vi "test Basic Future Resolution - Error.vi"(8 "error in (no error)":errorcluster, 11 "TestCase in":refnum<class "Futures Tests.lvclass">) -> (0 "error out":errorcluster, 3 "TestCase out":refnum<class "Futures Tests.lvclass">)   [LabVIEW 2017, in "Futures Tests.lvclass"]
uses:
  Futures Tests.lvclass
  <vilib>/Utility/error.llb/Error Cluster From Error Code.vi
  <vilib>/ErrorRing/Error Ring.xnode
  <vilib>/addons/_JKI Toolkits/VI Tester/TestCase.llb/TestCase.lvclass
  Futures/Futures.lvlib
  Futures/Future/Future.lvclass
  Futures/Promise/Promise.lvclass
  C:/Program Files (x86)/National Instruments/LabVIEW 2017/vi.lib/addons/_JKI Toolkits/VI Tester/TestCase.llb/TestCase.lvclass
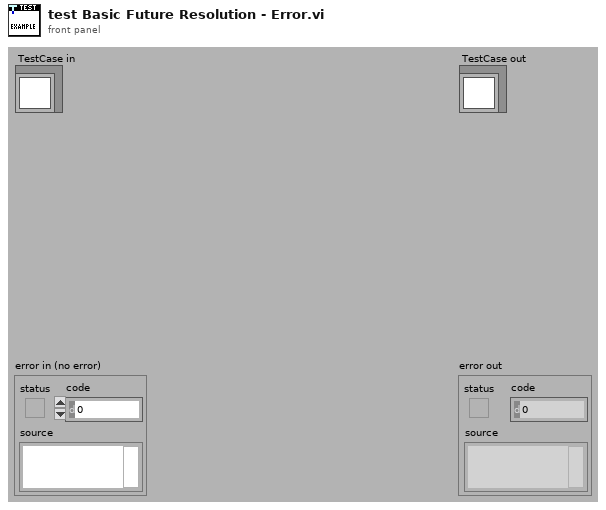
[diagram p1: front panel]
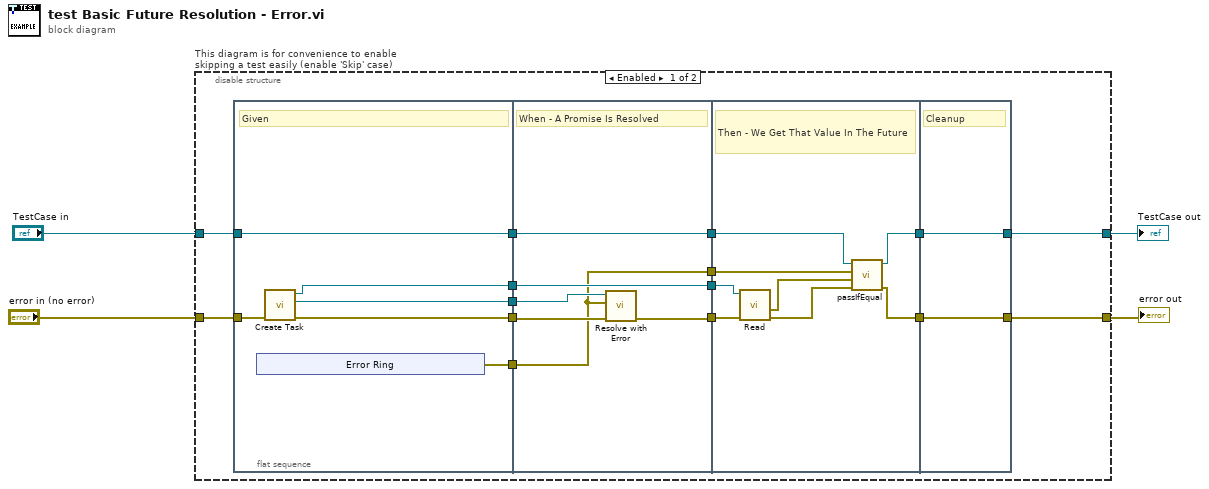
[diagram p0: block diagram]
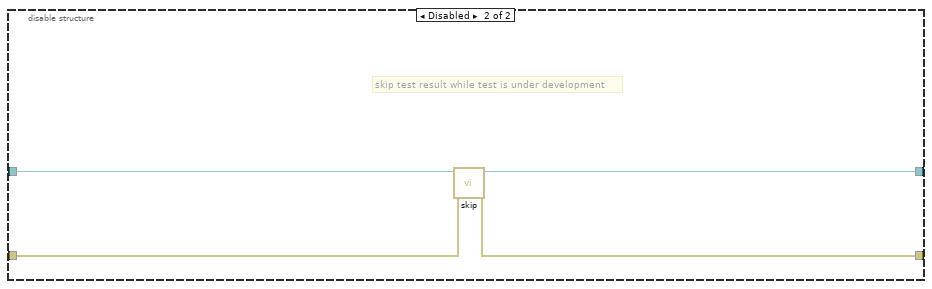
[diagram p2: hidden frame]
diagram:
  n1 = disable-structure "This diagram is for convenience to enable skipping a test easily (enable 'Skip' case)" shown="Enabled" {
    disable-tunnel: "TestCase in" -> [w13 w49]
    disable-tunnel: [w11 w47] -> w1
    disable-tunnel: [w10 w48] -> w3
    disable-tunnel: "error in (no error)" -> [w12 w46]
    frame Enabled {
      n2 = flat-sequence {
        tunnel: w12 -> [w24]
        tunnel: w13 -> [w25]
        tunnel: [w25] -> w19
        tunnel: [w23] -> w18
        tunnel: [w22] -> w9
        tunnel: [w21] -> w7
        tunnel: [w20] -> w5
        tunnel: [w35] -> w17
        tunnel: [w33] -> w16
        tunnel: w19 -> [w35]
        tunnel: w18 -> [w34]
        tunnel: w9 -> [w32]
        tunnel: [w31] -> w8
        tunnel: w7 -> [w31]
        tunnel: [w30] -> w6
        tunnel: w5 -> [w30]
        tunnel: [w42] -> w15
        tunnel: [w41] -> w14
        tunnel: w17 -> [w43]
        tunnel: w16 -> [w40]
        tunnel: w8 -> [w39]
        tunnel: w6 -> [w38]
        tunnel: [w44] -> w10
        tunnel: [w45] -> w11
        tunnel: w15 -> [w45]
        tunnel: w14 -> [w44]
        frame #0 {
          # "Given"
          n3 = xnode "Error Ring"() -> ("error out"=w20:errorcluster)
          n4 = call "Create Task.vi"("error in (no error)"=w24) -> ("error out"=w23:errorcluster, "Promise out"=w22:refnum<class "Promise.lvclass">, "Future out"=w21:refnum<class "Future.lvclass">)  [unwired: 8 in]
        }
        frame #1 {
          # "When - A Promise Is Resolved"
          n5 = call "Resolve with Error.vi"("error in (no error)"=w34, "Result"=w30, "Promise in"=w32) -> ("error out"=w33:errorcluster)  [unwired: 8 in]
        }
        frame #2 {
          # "Then - We Get That Value In The Future"
          n6 = call "Read.vi"("error in (no error)"=w40, "Future in"=w39) -> ("error out"=w37:errorcluster, "result error"=w36:errorcluster)  [unwired: 6 in, 2 out]
          n7 = call-dynamic "passIfEqual.vi"("error in (no error)"=w37, "y"=w36, "x"=w38, "TestCase in"=w43) -> ("error out"=w41:errorcluster, "TestCase out"=w42:refnum<class "Futures Tests.lvclass">)  [unwired: 6 in]
        }
        frame #3 {
          # "Cleanup"
        }
      }
    }
    frame Disabled {
      # "skip test result while test is under development"
      n8 = call <vilib>:"skip.vi"("error in (no error)"=w46, "TestCase in"=w49) -> ("error out"=w48:errorcluster, "TestCase out"=w47:refnum<class "Futures Tests.lvclass">)  [unwired: 8 in]
    }
  }
  "error out" <- w3
  "TestCase out" <- w1
